vi "Schließen.vi"(8 "Error In":errorcluster caption="Fehler (Eingang)", 11 "connection_ID_In":refnum<k5>) -> (0 "Error Out":errorcluster caption="Fehler (Ausgang)")   [LabVIEW 2019, in "Motor Treiber.lvlib"]
uses:
  Motor Treiber.lvlib
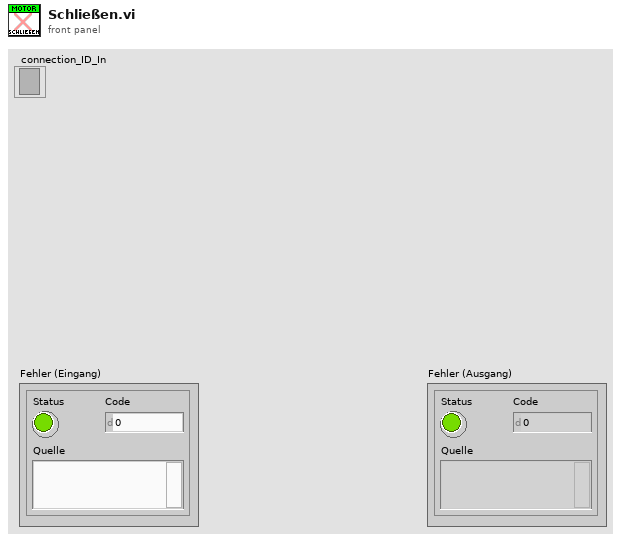
[diagram p1: front panel]
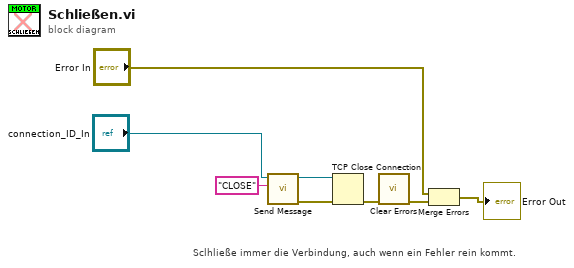
[diagram p0: block diagram]
diagram:
  # "Sclhließe immer die Verbindung, auch wenn ein Fehler rein kommt."
  n1 = call "Send Message.vi"("Nachricht"="CLOSE", "connection_ID_In"="connection_ID_In") -> ("Error Out"=w5:errorcluster, "connection_ID_Out"=w6:refnum<k5>)  [unwired: 8 in]
  n2 = TCP Close Connection(connection ID=w6, error in (no error)=w5) -> (error out=w8:errorcluster)  [unwired: 1 in, 1 out]
  n3 = call <vilib>:"Clear Errors.vi"("error in (no error)"=w8) -> ("error out"=w1:errorcluster)  [unwired: 5 in, 1 out]
  n4 = Merge Errors("Error In", w1) -> (→"Error Out":errorcluster)
